vi "Check if Icon Specified.vi"(1 "Device Icon Name":string[](array[string])) -> (0 "No Icon Specified":bool)   [LabVIEW 2014]
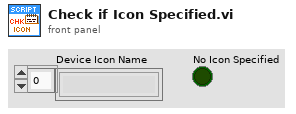
[diagram p1: front panel]
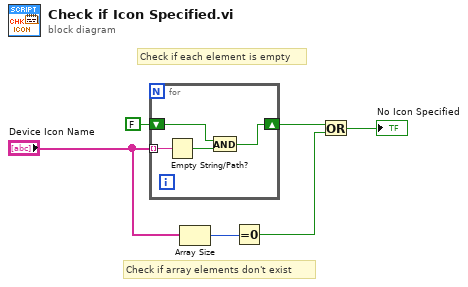
[diagram p0: block diagram]
diagram:
  # "Check if each element is empty"
  # "Check if array elements don't exist"
  n1 = for {
    tunnel: "Device Icon Name" -> [w10] mode=indexing
    shift-right: [w7] -> w3
    shift-left: FALSE -> [w8]
    n2 = Empty String/Path?(string/path=w10) -> (empty?=w9:bool)
    n3 = And(x=w8, y=w9) -> (x .and. y?=w7:bool)
  }
  n4 = Array Size(array="Device Icon Name") -> (size(s)=w4:i32)
  n5 = Equal To 0?(x=w4) -> (x = 0?=w2:bool)
  n6 = Or(x=w3, y=w2) -> (x .or. y?=→"No Icon Specified":bool)
